vi "PXI-Set Skip Samples.vi"(0 "Number of samples to skip (-1)":i32=-1, 11 "error in (no error)":errorcluster) -> (15 "error out":errorcluster)   [LabVIEW 2020]
uses:
  DAQ Engine VIs/PXI Globals.vi
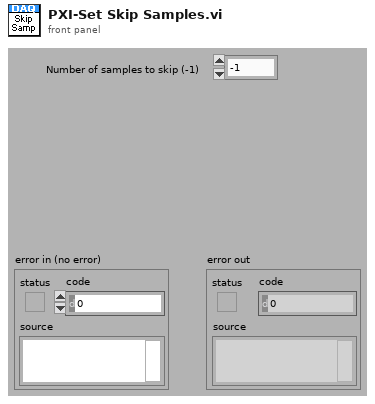
[diagram p1: front panel]
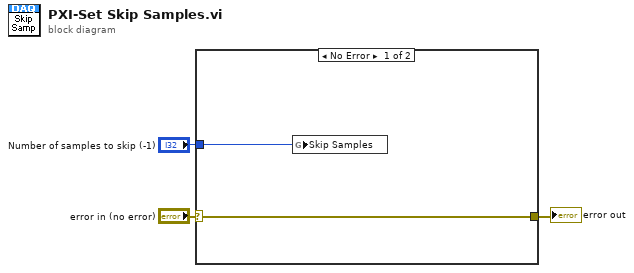
[diagram p0: block diagram]
diagram:
  n1 = case shown="No Error" "error in (no error)" {
    selector: "error in (no error)" -> [w5 w6]
    tunnel: "Number of samples to skip (-1)" -> [w4 _]
    tunnel: [w5 w6] -> w1
    frame No Error {
      n2 = global write "PXI Globals.vi" "Skip Samples"(w4) -> ()
    }
    frame Error {
    }
  }
  "error out" <- w1
